vi "getSalCommunicatorDL.vi"(8 "error in (no error)":errorcluster, 11 "MiddlewareSALThisComponent in":refnum<class "MiddlewareSALThisComponent.lvclass">) -> (0 "error out":errorcluster, 2 "SALCommunicatorDL.lvclass":refnum<class "SALCommunicatorDL.lvclass">, 3 "MiddlewareSALThisComponent out":refnum<class "MiddlewareSALThisComponent.lvclass">)   [LabVIEW 2016]
uses:
  MiddlewareSALThisComponent.lvclass
  home/andres/ct_cmpuserevents/ComponentTemplateCore/ComponentModel/ComponentModel/MiddlewareSAL/MiddlewareSAL.lvclass
  home/andres/ct_cmpuserevents/ComponentTemplateCore/ComponentModel/ComponentModel/Middleware/Middleware.lvclass
  SALCommunicatorDL/SALCommunicatorDL.lvclass
  home/andres/ct_cmpuserevents/SALCommunicatorTC/SALCommunicatorTC.lvclass
  home/andres/ct_cmpuserevents/SALCommunicator/SALCommunicator.lvclass
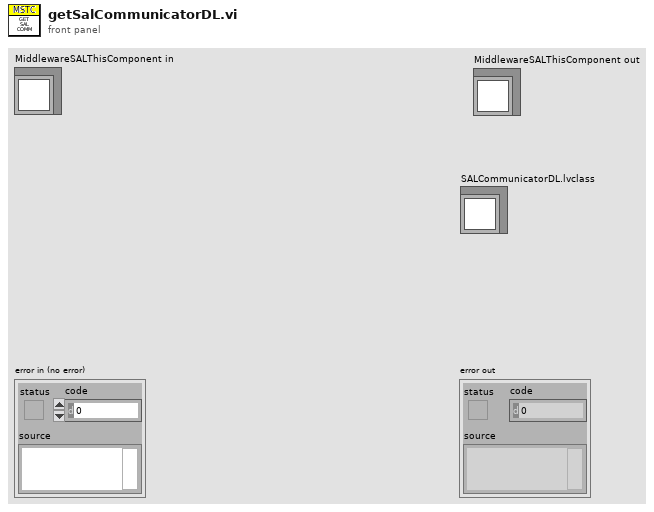
[diagram p1: front panel]
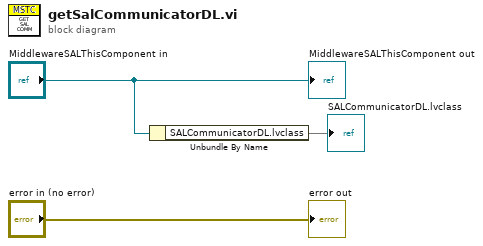
[diagram p0: block diagram]
diagram:
  n1 = Unbundle By Name("MiddlewareSALThisComponent in") -> ("SALCommunicatorDL.lvclass"=→"SALCommunicatorDL.lvclass")
  "error out" <- "error in (no error)"
  "MiddlewareSALThisComponent out" <- "MiddlewareSALThisComponent in"
